vi "CTSub.vi"(4 "GPU?":bool=TRUE, 6 "ROI?":bool, 8 "Segment Setup":T1={"threshold"=2.5e-08, "Depth"=1.0, "Remove Size "=25}, 9 "CSRsetup":T2={"SrcWidth"=768, "Angles"=336, "AngleStep"=0.84, "RotateCenter"=367, "SDDistance"=3500.0} {"SDDistance" format="%#.6g"; "AngleStep" format="%#_4f"}, 10 "ROIsetup":cluster{"SmallSize":i32, "Thresh":i32}={"SmallSize"=50, "Thresh"=0}, 11 "Image Pixels (U16)":u16[][](array[numeric])) -> (0 "nTiller":i32, 1 "watershed":i16[][](array[numeric]), 2 "ROIData":sgl[][](array[numeric]), 3 "Sinogram":i32[][](array[numeric]))   [LabVIEW 2015]
uses:
  fanROI.dll
  watershed.dll
  GrayReconstruct.dll
  MorphologicProcessing.dll
  LocalAreaWHR.dll
  CTTexture.dll
panel:
  in  "ErodeDepth":i32
  in  "WHRThreshold":dbl=1.2
  in  "AreaThrshold":i32=50
  out "End":i32
  out "Start":i32
  out "RotateAngle":i32
  out "ROIRect":i32[](array[numeric])
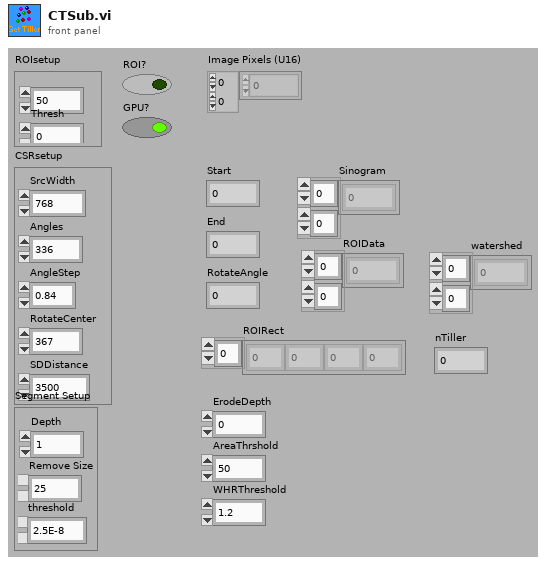
[diagram p1: front panel]
types:
  T1 = cluster{"threshold":sgl, "Depth":sgl, "Remove Size ":i32}
  T2 = cluster{"SrcWidth":i32, "Angles":i32, "AngleStep":sgl, "RotateCenter":i32, "SDDistance":sgl}
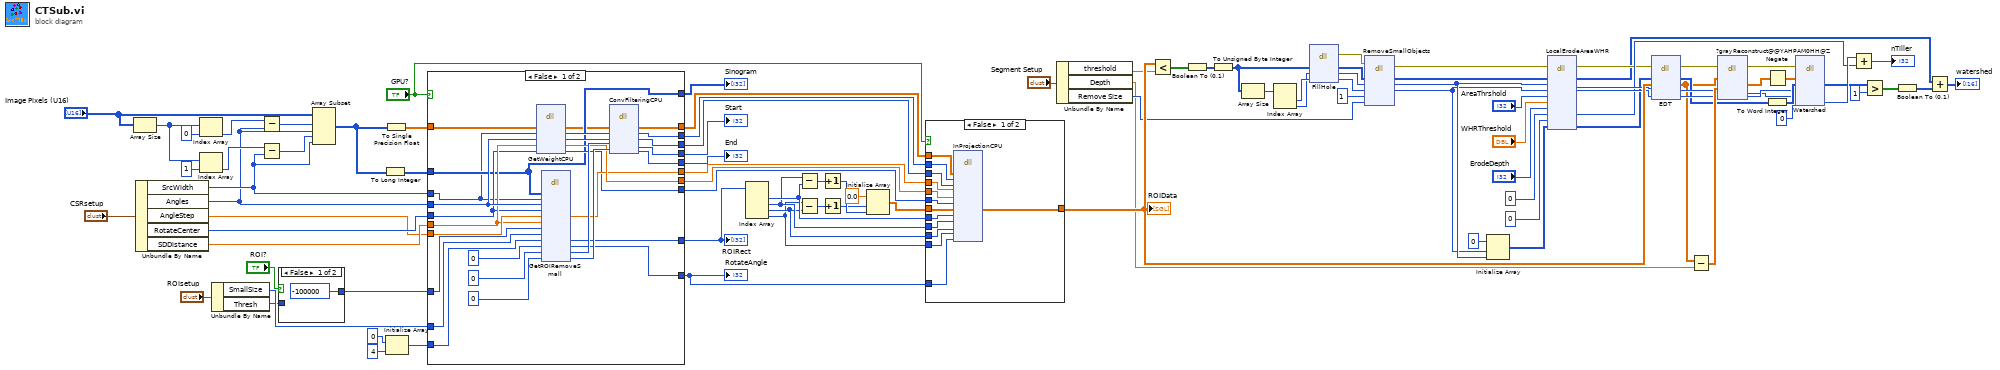
[diagram p0: block diagram]
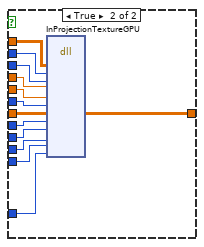
[diagram p2: hidden frame]
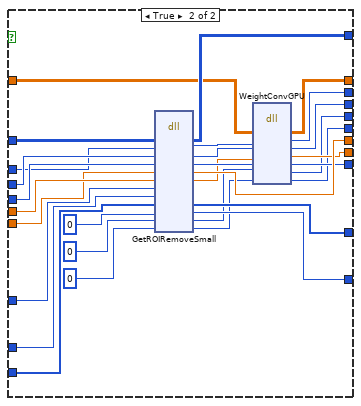
[diagram p3: hidden frame]
diagram:
  n1 = Array Size(array="Image Pixels (U16)") -> (size(s)=w10:i32[])
  n2 = Unbundle By Name("CSRsetup") -> ("SrcWidth"=w6:i32, "Angles"=w5:i32, "AngleStep"=w81:sgl, "RotateCenter"=w99:i32, "SDDistance"=w98:sgl)
  n3 = Index Array(array=w10, index=0) -> (element=w9:i32)
  n4 = Index Array(array=w10, index=1) -> (element=w7:i32)
  n5 = Unbundle By Name("ROIsetup") -> ("SmallSize"=w49:i32, "Thresh"=w43:i32)
  n6 = Subtract(x=w9, y=w5) -> (x-y=w13:i32)
  n7 = Subtract(x=w7, y=w6) -> (x-y=w12:i32)
  n8 = case shown="False" "ROI?" {
    tunnel: [-100000 ("Thresh") w102] -> w42
    tunnel: w43 -> [_ w102]
    frame False {
    }
    frame True {
    }
  }
  n9 = Array Subset(array="Image Pixels (U16)", index (row)=w13, length (row)=w5, index (col)=w12, length (col)=w6) -> (w4:u16[][])
  n10 = To Long Integer(number=w4) -> (32bit integer=w14:i32[][])
  n11 = To Single Precision Float(number=w4) -> (single precision float=w1:sgl[][])
  n12 = Initialize Array(0 ("element"), 4 ("dimension size")) -> (w95:i32[])
  n13 = case shown="False" "GPU?" {
    tunnel: w1 -> [w123 w131]
    tunnel: [w122 w160] -> w2
    tunnel: w5 -> [w111 w159]
    tunnel: w99 -> [w109 w158]
    tunnel: w98 -> [w110 w157]
    tunnel: w95 -> [w118 w156]
    tunnel: [w113 w155] -> w94
    tunnel: [w112 w154] -> w93
    tunnel: [w107 w153] -> w92
    tunnel: [w108 w152] -> w91
    tunnel: [w106 w151] -> w90
    tunnel: w81 -> [w121 w150]
    tunnel: [w117 w149] -> w80
    tunnel: [w115 w148] -> w77
    tunnel: [w114 w147] -> w76
    tunnel: [w116 w146] -> w75
    tunnel: [w105 w132] -> w74
    tunnel: w49 -> [w119 w145]
    tunnel: w42 -> [w120 w144]
    tunnel: w6 -> [w103 w134]
    tunnel: w14 -> [w105 w133]
    frame False {
      n14 = dll-call lib="PTH2jabs E文章投稿&51. 代明球老师-玉米胁迫实验CT程序断层重建程序\nCTTexture.dll" fn="GetWeightCPU" label="WeightCPU"("Sinogram"=w123, "Width"=w103, "Angles"=w111, "SDDistance"=w110, "RotateCenter"=w109) -> ("Sinogram"=w104:sgl[][], "Width"=w129:i32, "Angles"=w130:i32, "SDDistance"=w108:sgl, "RotateCenter"=w106:i32)  [unwired: 3 in, 3 out]
      n15 = dll-call lib="PTH2gabs E文章投稿&51. 代明球老师-玉米胁迫实验CT程序断层重建程序\nfanROI.dll" fn="GetROIRemoveSmall" label="ROI"("Sinogram"=w105, "Width"=w103, "Angles"=w111, "RotateCenter"=w109, "AngleStep"=w121, "SDistance"=w110, "Thresh"=w120, "SmallSize"=w119, "ROIRect"=w118, "RotateAngle"=0, "Start"=0, "End"=0) -> ("AngleStep"=w107:sgl, "ROIRect"=w117:i32[], "RotateAngle"=w116:i32, "Start"=w125:i32, "End"=w124:i32)  [unwired: 9 in, 4 out]
      n16 = dll-call lib="PTH2jabs E文章投稿&51. 代明球老师-玉米胁迫实验CT程序断层重建程序\nCTTexture.dll" fn="ConvFilteringCPU" label="ConvCPU"("Sinogram"=w104, "Width"=w129, "Angles"=w130, "Start"=w125, "End"=w124) -> ("Sinogram"=w122:sgl[][], "Width"=w113:i32, "Angles"=w112:i32, "Start"=w115:i32, "End"=w114:i32)  [unwired: 3 in, 3 out]
    }
    frame True {
      n17 = dll-call lib="PTH2gabs E文章投稿&51. 代明球老师-玉米胁迫实验CT程序断层重建程序\nfanROI.dll" fn="GetROIRemoveSmall" label="ROI"("Sinogram"=w133, "Width"=w134, "Angles"=w159, "RotateCenter"=w158, "AngleStep"=w150, "SDistance"=w157, "Thresh"=w144, "SmallSize"=w145, "ROIRect"=w156, "RotateAngle"=0, "Start"=0, "End"=0) -> ("Sinogram"=w132:i32[][], "Width"=w136:i32, "Angles"=w137:i32, "RotateCenter"=w138:i32, "AngleStep"=w153:sgl, "SDistance"=w135:sgl, "ROIRect"=w149:i32[], "RotateAngle"=w146:i32, "Start"=w140:i32, "End"=w139:i32)  [unwired: 5 in, 3 out]
      n18 = dll-call lib="PTH2jabs E文章投稿&51. 代明球老师-玉米胁迫实验CT程序断层重建程序\nCTTexture.dll" fn="WeightConvGPU" label="ConvGPU"("Sinogram"=w131, "Width"=w136, "Angles"=w137, "SDDistance"=w135, "RotateCenter"=w138, "Start"=w140, "End"=w139) -> ("Sinogram"=w160:sgl[][], "Width"=w155:i32, "Angles"=w154:i32, "SDDistance"=w152:sgl, "RotateCenter"=w151:i32, "Start"=w148:i32, "End"=w147:i32)  [unwired: 3 in, 3 out]
    }
  }
  "ROIRect" <- w80
  "RotateAngle" <- w75
  "Start" <- w77
  "End" <- w76
  "Sinogram" <- w74
  n19 = Index Array(array=w80) -> (element #1=w85:i32, element #2=w84:i32, element #3=w83:i32, element #4=w82:i32)  [unwired: 4 in]
  n20 = Subtract(x=w84, y=w85) -> (x-y=w87:i32)
  n21 = Subtract(x=w82, y=w83) -> (x-y=w88:i32)
  n22 = Increment(x=w87) -> (x+1=w79:i32)
  n23 = Increment(x=w88) -> (x+1=w78:i32)
  n24 = Initialize Array(sgl 0.0 ("element"), w78, w79) -> (w86:sgl[][])
  n25 = case shown="False" "GPU?" {
    tunnel: w2 -> [w173 w186]
    tunnel: w94 -> [w172 w185]
    tunnel: w93 -> [w171 w184]
    tunnel: w92 -> [w170 w183]
    tunnel: w91 -> [w169 w182]
    tunnel: w90 -> [w168 w181]
    tunnel: w86 -> [w167 w180]
    tunnel: w85 -> [w166 w179]
    tunnel: w84 -> [w165 w178]
    tunnel: w83 -> [w164 w177]
    tunnel: w82 -> [w163 w176]
    tunnel: w75 -> [w162 w175]
    tunnel: [w161 w174] -> w51
    frame False {
      n26 = dll-call lib="PTH2jabs E文章投稿&51. 代明球老师-玉米胁迫实验CT程序断层重建程序\nCTTexture.dll" fn="InProjectionCPU" label="InProjection"("Sinogram"=w173, "Width"=w172, "Angles"=w171, "AngleStep"=w170, "SDistance"=w169, "RotateCenter"=w168, "ROIData"=w167, "xmin"=w166, "xmax"=w165, "ymin"=w164, "ymax"=w163, "RotateAngle"=w162) -> ("ROIData"=w161:sgl[][])  [unwired: 14 in, 3 out]
    }
    frame True {
      n27 = dll-call lib="PTH2jabs E文章投稿&51. 代明球老师-玉米胁迫实验CT程序断层重建程序\nCTTexture.dll" fn="InProjectionTextureGPU" label="InProjection"("Sinogram"=w186, "Width"=w185, "Angles"=w184, "AngleStep"=w183, "SDistance"=w182, "RotateCenter"=w181, "ROIData"=w180, "xmin"=w179, "xmax"=w178, "ymin"=w177, "ymax"=w176, "RotateAngle"=w175) -> ("ROIData"=w174:sgl[][])  [unwired: 14 in, 3 out]
    }
  }
  "ROIData" <- w51
  n28 = Unbundle By Name("Segment Setup") -> ("threshold"=w47:sgl, "Depth"=w45:sgl, "Remove Size"=w46:i32)
  n29 = Less?(x=w51, y=w47) -> (x < y?=w73:bool[][])
  n30 = Boolean To (0,1)(Boolean=w73) -> (0, 1=w61:i16[][])
  n31 = To Unsigned Byte Integer(number=w61) -> (unsigned 8bit integer=w58:u8[][])
  n32 = Array Size(array=w58) -> (size(s)=w65:i32[])
  n33 = Index Array(array=w65) -> (element #1=w56:i32, element #2=w52:i32)  [unwired: 2 in]
  n34 = dll-call lib="PTH2vabs E文章投稿&51. 代明球老师-玉米胁迫实验CT程序断层重建程序MorphologicProcessing.dll" fn="FillHole"("BWArrayOrg"=w58, "Width"=w52, "Height"=w56) -> (error out=w30:errorcluster, "BWArrayOrg"=w57:u8[][], "Width"=w54:u32, "Height"=w53:u32)  [unwired: 3 in, 2 out]
  n35 = dll-call lib="PTH2vabs E文章投稿&51. 代明球老师-玉米胁迫实验CT程序断层重建程序MorphologicProcessing.dll" fn="RemoveSmallObjects"(error in=w30, "BWArray"=w57, "Width"=w54, "Height"=w53, "targetPixel"=u8 1, "SmallSize"=w46) -> (error out=w31:errorcluster, "BWArray"=w40:u8[][], "Width"=w27:u32, "Height"=w26:u32)  [unwired: 4 in, 2 out]
  n36 = Initialize Array(u8 0 ("element"), w26, w27) -> (w25:u8[][])
  n37 = dll-call lib="PTH2mabs E文章投稿&51. 代明球老师-玉米胁迫实验CT程序断层重建程序LocalAreaWHR.dll" fn="LocalErodeAreaWHR"(error in=w31, "BWData"=w40, "BWWidth"=w27, "BWHeight"=w26, "AreaThrshold"="AreaThrshold", "WHRThreshold"="WHRThreshold", "ErodeDepth"="ErodeDepth", "nAreaRemove"=0 ("totalArea"), "nAreaRemaining"=0 ("nAreaRemove"), "BWArray"=w25) -> (error out=w17:errorcluster, "BWData"=w16:u8[][], "BWWidth"=w34:i32, "BWHeight"=w33:i32, "nAreaRemove"=w22:i32, "BWArray"=w24:u8[][])  [unwired: 5 in, 3 out]
  n38 = dll-call lib="PTH2vabs E文章投稿&51. 代明球老师-玉米胁迫实验CT程序断层重建程序MorphologicProcessing.dll" fn="EDT"(error in=w17, "data"=w24, "Dst-data"=w51, "width"=w34, "height"=w33) -> (error out=w68:errorcluster, "data"=w64:u8[][], "Dst-data"=w62:sgl[][], "width"=w71:i32, "height"=w70:i32)  [unwired: 2 in, 2 out]
  n39 = Subtract(x=w62, y=w45) -> (x-y=w72:sgl[][])
  n40 = dll-call lib="PTH2pabs E文章投稿&51. 代明球老师-玉米胁迫实验CT程序断层重建程序GrayReconstruct.dll" fn="?grayReconstruct@@YAHPAM0HH@Z" label="GrayRcst"(error in=w68, "MaskI"=w62, "MarkerJ"=w72, "width"=w71, "height"=w70) -> (error out=w67:errorcluster, "MarkerJ"=w69:sgl[][], "width"=w59:i32, "height"=w60:i32)  [unwired: 3 in, 2 out]
  n41 = Negate(x=w69) -> (-x=w66:sgl[][])
  n42 = To Word Integer(number=w64) -> (16bit integer=w63:i16[][])
  n43 = dll-call lib="PTH2jabs E文章投稿&51. 代明球老师-玉米胁迫实验CT程序断层重建程序\nwatershed.dll" fn="Watershed"(error in=w67, "rice"=w66, "watershed"=w63, "width"=w60, "height"=w59, "NCatchment"=0) -> ("watershed"=w19:i16[][], "NCatchment"=w23:i32)  [unwired: 5 in, 3 out]
  n44 = Add(x=w23, y=w22) -> (x+y=→"nTiller":i32)
  n45 = Greater?(x=w19, y=i16 1 ("nAreaRemove")) -> (0:w29:bool[][])
  n46 = Boolean To (0,1)(Boolean=w29) -> (0, 1=w18:i16[][])
  n47 = Add(x=w16, y=w18) -> (x+y=→"watershed":i16[][])
